vi "Simulation Configuration Read If Present.vi"(8 "error in (no error)":errorcluster, 10 "configuration":path=path "simulation configuration.ini", 11 "simulation configuration":T1={"maxTime"=5.0, "enableVisualization"=TRUE, "Environment Definition"=path "iRobot Navigation State Machine.vi", "Record Location"=path "Simulation Record.xml", "autograde?"=TRUE, "interactive?"=FALSE, "Feedback Mode"=enum."debug navigation", "Robot State Charts"=[path "C:/Users/blueuser/Desktop/Robo Sim Berkley/cpsgrader-release-0.4/Simulators/EECS149lab/src/LabVIEW/statechart/Simulation Statechart.vi"], "statechart"=path "C:/Users/blueuser/Desktop/Robo Sim Berkley/cpsgrader-release-0.4/Simulators/EECS149lab/src/LabVIEW/statechart/Simulation Statechart.vi"}) -> (0 "error out":errorcluster, 3 "simulation configuration":T1={"maxTime"=5.0, "enableVisualization"=TRUE, "Environment Definition"=path "iRobot Navigation State Machine.vi", "Record Location"=path "Simulation Record.xml", "autograde?"=TRUE, "interactive?"=FALSE, "Feedback Mode"=enum."debug navigation", "Robot State Charts"=[path "C:/Users/blueuser/Desktop/Robo Sim Berkley/cpsgrader-release-0.4/Simulators/EECS149lab/src/LabVIEW/statechart/Simulation Statechart.vi"], "statechart"=path "C:/Users/blueuser/Desktop/Robo Sim Berkley/cpsgrader-release-0.4/Simulators/EECS149lab/src/LabVIEW/statechart/Simulation Statechart.vi"})   [LabVIEW 2015]
uses:
  CyberSim interface/Simulation Configuration.ctl
  autograder/feedbackMode.ctl
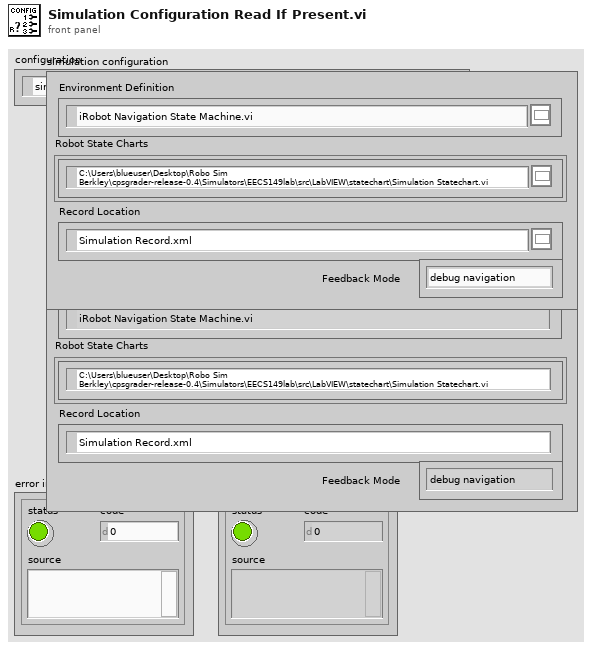
[diagram p1: front panel]
types:
  T1 = typedef "Simulation Configuration.ctl" = cluster{"maxTime":sgl, "enableVisualization":bool, "Environment Definition":path, "Record Location":path, "autograde?":bool, "interactive?":bool, "Feedback Mode":T2, "Robot State Charts":path[], "statechart":path}
  T2 = typedef "feedbackMode.ctl" = enum32{"debug navigation", "debug hill climb", "autograde navigation", "autograde hill climb"}
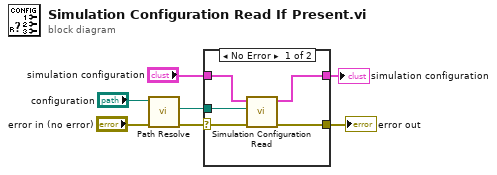
[diagram p0: block diagram]
diagram:
  n1 = call "Path Resolve.vi"("Error In"="error in (no error)", "absolute or relative path"="configuration") -> ("Error Out"=w5:errorcluster, "resolved path"=w3:path)  [unwired: 8 in]
  n2 = case shown="No Error" w5 {
    selector: w5 -> [w11 _]
    tunnel: "simulation configuration" -> [w12 w13]
    tunnel: w3 -> [w10 _]
    tunnel: [w9 _] -> w2
    tunnel: [w8 w13] -> w1
    frame No Error {
      n3 = call "Simulation Configuration Read.vi"("error in (no error)"=w11, "configuration"=w10, "simulation configuration"=w12) -> ("error out"=w9:errorcluster, "simulation configuration"=w8:T1)  [unwired: 7 in]
    }
    frame Error {
    }
  }
  "error out" <- w2
  "simulation configuration" <- w1
